vi "Get global var.vi"(8 "error in (no error)":errorcluster, 10 "Key Name":string="test_pc_name", 11 "Section Name":string="general") -> (0 "error out":errorcluster, 1 "Yes?":bool, 2 "KeyFound?":bool, 3 "Key data from file":string)   [LabVIEW 2013]
doc: "Gets key data from global.ini file in exe directory"
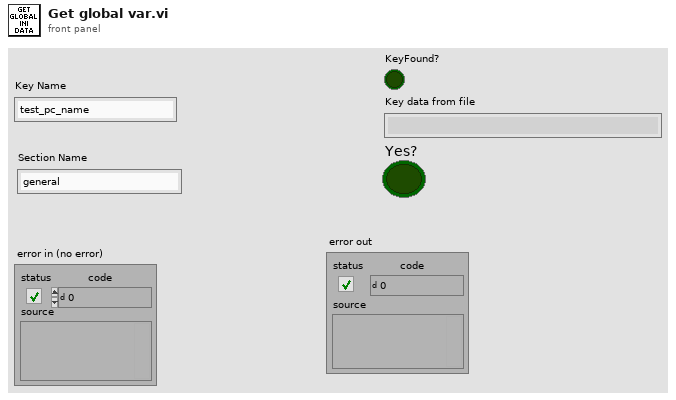
[diagram p1: front panel]
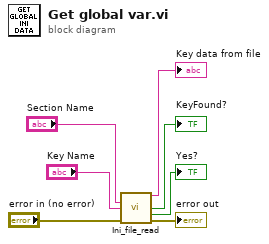
[diagram p0: block diagram]
diagram:
  n1 = call "Ini_file_read.vi"("Section Name"="Section Name", "Key Name"="Key Name", "error in (no error)"="error in (no error)") -> ("Key data"=→"Key data from file":string, "KeyFound?"=→"KeyFound?":bool, "Yes?"=→"Yes?":bool, "error out"=→"error out":errorcluster)  [unwired: 9 in]
